vi "HeatingRate.vi"() -> ()   [LabVIEW 2012]
uses:
  <vilib>/Utility/error.llb/DialogType.ctl
  <vilib>/DAQmx/write.llb/DAQmx Write (Digital Wfm 1Chan NSamp).vi
  <vilib>/DAQmx/read.llb/DAQmx Read (Counter 1D U32 1Chan NSamp).vi
  <vilib>/DAQmx/create/channels.llb/DAQmx Create Channel (CI-Count Edges).vi
  <vilib>/DAQmx/create/channels.llb/DAQmx Create Channel (DO-Digital Output).vi
  <vilib>/DAQmx/create/channels.llb/DAQmx Create Channel (CO-Pulse Generation-Frequency).vi
  <vilib>/DAQmx/configure/timing.llb/DAQmx Timing (Implicit).vi
  <vilib>/Waveform/DWDTOps.llb/Digital Pattern Generator (Single Value).vi
  <vilib>/Waveform/DWDTOps.llb/DWDT Append Digital Samples.vi
  <vilib>/Waveform/DWDTOps.llb/DWDT Append Digital Signals.vi
  <vilib>/Waveform/DWDTOps.llb/DWDT Digital Size.vi
  <vilib>/DAQmx/configure/timing.llb/DAQmx Timing (Sample Clock).vi
  <vilib>/Waveform/DWDTOps.llb/DWDT Invert Digital.vi
  <vilib>/Waveform/DWDTOps.llb/DWDT Uncompress Digital.vi
  <vilib>/DAQmx/miscellaneous.llb/DAQmx Fill In Error Info.vi
  <resource>/objmgr/daqmx.rc
panel:
  in  "Mechanical Shutter":bool
  in  "Threshold":u32
  in  "Recool Time (ms)":u32=1000
  out "Run No":i32=16
  in  "Clock Rate":dbl=10000.0
  in  "Off Time (s)":dbl=0.5
  out "Waveform Graph":u32[](graph)=[0, 0, 0, 0, 0, 0, 0, 0, 0, 0, 0, 0, 0, 0, 0, 0, 0, 0, 0, 0, 0, 0, 0, 0, 0, 0, 0, 0, 0, 0, 0, 0, 0, 0, 0, 0, 0, 0, 0, 0, 0, 0, 0, 0, 0, 0, 0, 0, 0, 0, 0, 0, 0, 0, 0, 0, 0, 0, 0, 0, 0, 0, 0, 0, 0, 0, 0, 0, 0, 0, 0, 0, 0, 0, 0, 0, 0, 0, 0, 0, 0, 0, 0, 0, 0, 0, 0, 0, 0, 0, 0, 0, 0, 0, 0, 0, 0, 0, 0, 0, 0, 0, 0, 0, 0, 0, 0, 0, 0, 0, 0, 0, 0, 0, 0, 0, 0, 0, 0, 0, 0, 0, 0, 0, 0, 0, 0, 0, 0, 0, 0, 0, 0, 0, 0, 0, 0, 0, 0, 0, 0, 0, 0, 0, 0, 0, 0, 0, 0, 0, 0, 0, 0, 0, 0, 0, 0, 0, 0, 0, 0, 0, 0, 0, 0, 0, 0, 0, 0, 0, 0, 0, 0, 0, 0, 0, 0, 0, 0, 0, 0, 0, 0, 0, 0, 0, 0, 0, 0, 0, 0, 0, 0, 0, 0, 0, 0, 0, 0, 0, 1, 1, 0, 0, 1, 0, 0, 0, 2, 3, 0, 0, 1, 3, 1, 2, 1, 2, 3, 0, 2, 2, 1, 1, 0, 1, 2, 0, 1, 1, 2, 2, 1, 1, 2, 1, 2, 0, 1, 1, 4, 0, 0, 1, 1, 0, 1, 0, 0, 0, 2, 0, 1, 0, 0, 1, 0, 0, 1, 0, 1, 1, 0, 1, 2, 0, 1, 1, 0, 1, 1, 1, 1, 2, 1, 0, 1, 0, 1, 1, 1, 1, 0, 1, 1, 1, 2, 1, 1, 1, 1, 0, 2, 0, 0, 0, 0, 3, 1, 2, 0, 1, 3, 0, 2, 1, 2, 2, 0, 1, 3, 1, 0, 1, 0, 3, 0, 3, 2, 0, 0, 4, 0, 0, 0, 1, 1, 3, 1, 0, 0, 1, 0, 0, 0, 0, 0, 0, 1, 1, 0, 1, 0, 0, 0, 1, 0, 0, 2, 0, 0, 1, 1, 1, 0, 1, 1, 0, 1, 1, 1, 2, 0, 0, 3, 1, 1, 0, 2, 0, 1, 0, 0, 1, 0, 3, 0, 4, 2, 1, 1, 1, 2, 1, 1, 1, 1, 1, 1, 0, 1, 0, 1, 1, 0, 1, 2, 0, 1]
  in  "Runs":i32=100
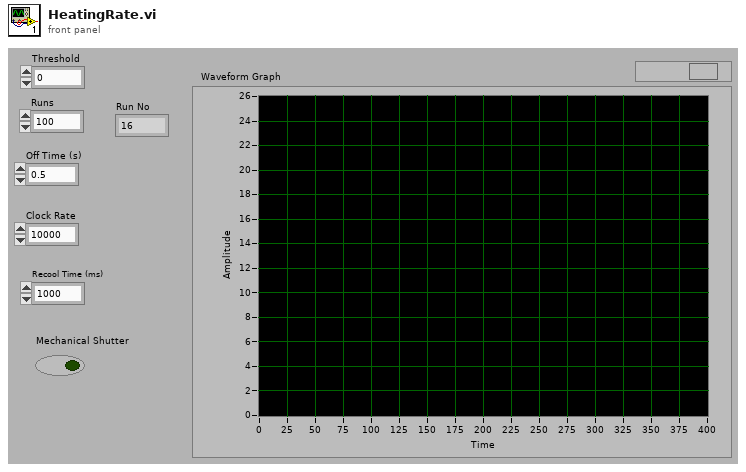
[diagram p1: front panel]
types:
  T1 = enum16{"open", "replace", "create", "open or create", "replace or create", "replace or create with confirmation"}
  T2 = typedef "DialogType.ctl" = u16
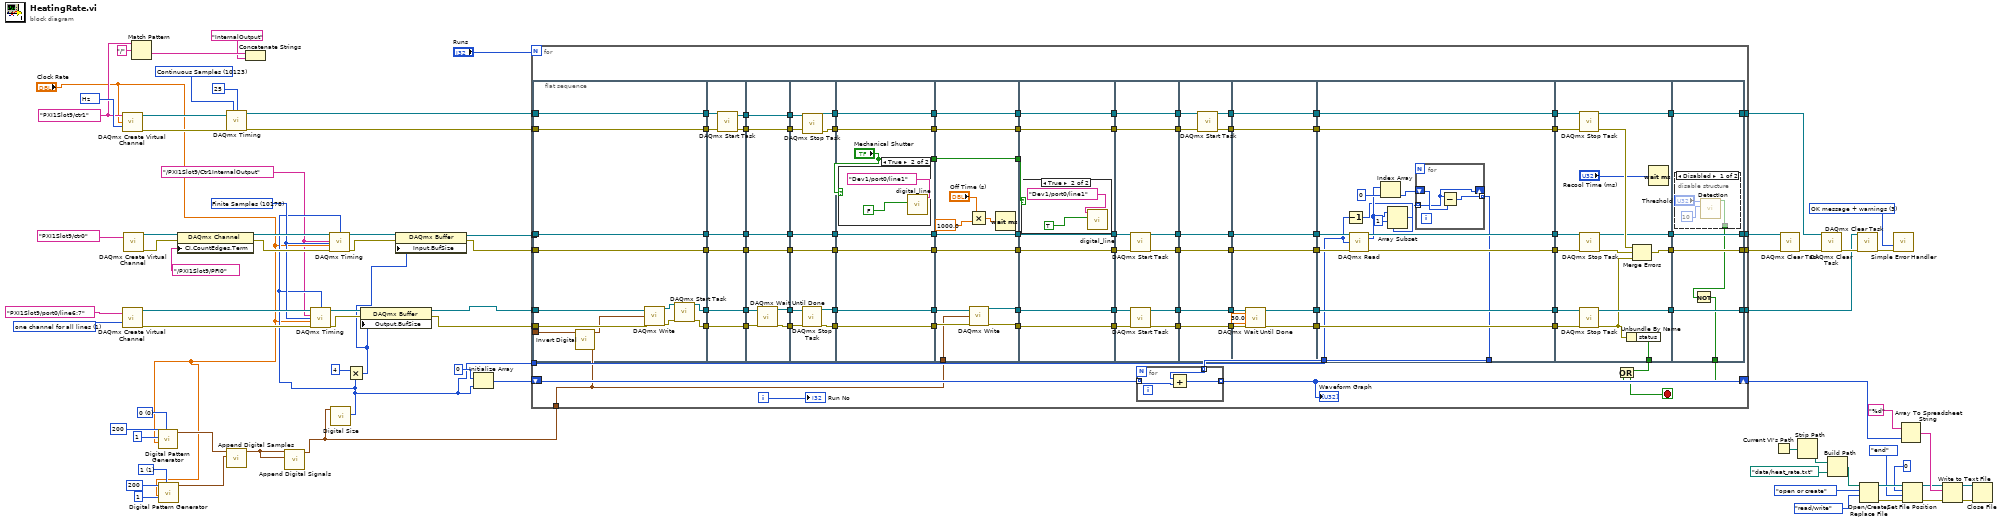
[diagram p0: block diagram]
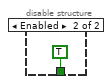
[diagram p4: hidden frame]
diagram:
  w3 = tag "/PXI1Slot9/Ctr1InternalOutput" ("source")
  w16 = u8 1 items=["0", "1", "Z", "L", "H", "X", "T", "V"] ("value")
  w17 = u8 0 items=["0", "1", "Z", "L", "H", "X", "T", "V"] ("value")
  w39 = 10178 items=["Finite Samples"=10178, "Continuous Samples"=10123, "Hardware Timed Single Point"=12522] ("sample mode")
  w52 = T2 3 items=["no dialog", "OK message", "continue or stop message", "OK message + warnings", "continue/stop + warnings"] ("type of dialog (OK msg:1)")
  w58 = 1 items=["one channel for each line", "one channel for all lines"] ("line grouping")
  w61 = tag "PXI1Slot9/ctr1" ("counter")
  w62 = 10373 items=["Hz"=10373] ("units")
  w56 = 10123 items=["Finite Samples"=10178, "Continuous Samples"=10123] ("sample mode")
  n1 = call-poly <vilib>:"DAQmx Create Virtual Channel.vi"("frequency"="Clock Rate", "counter"=w61, "units"=w62) -> ("task out"=w67:refnum<k21>, "error out"=w66:errorcluster)  [unwired: 11 in]
  n2 = call-poly <vilib>:"DAQmx Create Virtual Channel.vi"("lines"=tag "PXI1Slot9/port0/line6:7", "line grouping"=w58) -> ("task out"=w60:refnum<k21>, "error out"=w59:errorcluster)  [unwired: 12 in]
  n3 = call-poly <vilib>:"DAQmx Create Virtual Channel.vi"("counter"=tag "PXI1Slot9/ctr0") -> ("task out"=w70:refnum<k21>, "error out"=w69:errorcluster)  [unwired: 13 in]
  n4 = Match Pattern(string=w61, regular expression="/") -> (after substring=w64:string)  [unwired: 1 in, 3 out]
  n5 = call-poly <vilib>:"Digital Pattern Generator.vi"("value"=w17, "sample rate"="Clock Rate", "number of signals"=u32 1, "number of samples"=u32 200) -> ("digital waveform"=w12:digitalwaveform)  [unwired: 6 in, 1 out]
  n6 = call-poly <vilib>:"Digital Pattern Generator.vi"("value"=w16, "sample rate"="Clock Rate", "number of signals"=u32 1, "number of samples"=u32 200) -> ("digital waveform"=w11:digitalwaveform)  [unwired: 6 in, 1 out]
  n7 = property class="DAQmx Channel"(reference=w70, error in=w69, "CI.CountEdges.Term"=tag "/PXI1Slot9/PFI0") -> (reference out=w72:refnum<k21>, error out=w71:errorcluster)
  n8 = call-poly <vilib>:"DAQmx Timing.vi"("task/channels in"=w67, "sample mode"=w56, "samples per channel"=25, "error in"=w66) -> ("task out"=w2:refnum<k21>, "error out"=w1:errorcluster)  [unwired: 10 in]
  n9 = call-poly <vilib>:"Append Digital Samples.vi"("digital waveform B"=w11, "digital waveform A"=w12) -> ("digital waveform out"=w5:digitalwaveform)  [unwired: 8 in, 1 out]
  n10 = Concatenate Strings(w64, "InternalOutput" ("Local Terminal Name")) -> ()  [unwired: 1 out]
  n11 = call-poly <vilib>:"Append Digital Signals.vi"("digital waveform (low bits)"=w5, "digital waveform (high bits)"=w5) -> ("digital waveform out"=w4:digitalwaveform)  [unwired: 8 in, 1 out]
  n12 = call-poly <vilib>:"Digital Size.vi"("digital waveform in"=w4) -> ("number of samples"=w10:i32)  [unwired: 7 in, 3 out]
  n13 = call-poly <vilib>:"DAQmx Timing.vi"("task/channels in"=w60, "sample mode"=w39, "samples per channel"=w10, "rate"="Clock Rate", "source"=w3, "error in"=w59) -> ("task out"=w47:refnum<k21>, "error out"=w46:errorcluster)  [unwired: 8 in]
  n14 = call-poly <vilib>:"DAQmx Timing.vi"("task/channels in"=w72, "sample mode"=w39, "samples per channel"=w10, "rate"="Clock Rate", "source"=w3, "error in"=w71) -> ("task out"=w44:refnum<k21>, "error out"=w43:errorcluster)  [unwired: 8 in]
  n15 = Multiply(x=4, y=w10) -> (x*y=w18:i32)
  n16 = property class="DAQmx Buffer"(reference=w47, error in=w46, "Output.BufSize"=w18) -> (reference out=w8:refnum<k21>, error out=w7:errorcluster)
  n17 = property class="DAQmx Buffer"(reference=w44, error in=w43, "Input.BufSize"=w18) -> (reference out=w42:refnum<k21>, error out=w41:errorcluster)
  n18 = Initialize Array(0, w10) -> (w38:i32[])
  n19 = for {
    N: "Runs" -> [_]
    tunnel: w8 -> [w140]
    tunnel: w7 -> [w139]
    tunnel: w2 -> [w138]
    tunnel: w1 -> [w137]
    tunnel: [w136] -> w51
    tunnel: [w135] -> w50
    tunnel: [w134] -> w49
    tunnel: [w133] -> w48
    tunnel: w42 -> [w132]
    tunnel: w41 -> [w131]
    shift-right: [w128] -> w33
    shift-left: w38 -> [w130]
    tunnel: w10 -> [w127]
    tunnel: w4 -> [w107]
    i -> [w126]
    stop <- w76 stop-if-true
    n20 = flat-sequence {
      tunnel: w137 -> [w176]
      tunnel: w138 -> [w177]
      tunnel: w139 -> [w174]
      tunnel: w140 -> [w175]
      tunnel: w131 -> [w178]
      tunnel: w132 -> [w179]
      tunnel: [w179] -> w125
      tunnel: [w178] -> w124
      tunnel: [w170] -> w123
      tunnel: [w171] -> w122
      tunnel: [w177] -> w121
      tunnel: [w176] -> w120
      tunnel: w107 -> [w169]
      tunnel: w125 -> [w187]
      tunnel: [w187] -> w119
      tunnel: w124 -> [w186]
      tunnel: [w186] -> w117
      tunnel: w123 -> [w185]
      tunnel: [w185] -> w115
      tunnel: w122 -> [w184]
      tunnel: [w184] -> w113
      tunnel: w121 -> [w183]
      tunnel: w120 -> [w182]
      tunnel: [w181] -> w111
      tunnel: [w180] -> w110
      tunnel: w119 -> [w195]
      tunnel: [w195] -> w118
      tunnel: w117 -> [w194]
      tunnel: [w194] -> w116
      tunnel: w115 -> [w191]
      tunnel: [w190] -> w114
      tunnel: w113 -> [w188]
      tunnel: [w193] -> w112
      tunnel: w111 -> [w193]
      tunnel: w110 -> [w192]
      tunnel: [w192] -> w109
      tunnel: [w189] -> w108
      tunnel: w118 -> [w205]
      tunnel: [w205] -> w106
      tunnel: w116 -> [w204]
      tunnel: [w204] -> w104
      tunnel: w114 -> [w199]
      tunnel: [w196] -> w102
      tunnel: w112 -> [w203]
      tunnel: w109 -> [w202]
      tunnel: w108 -> [w198]
      tunnel: [w201] -> w100
      tunnel: [w200] -> w98
      tunnel: [w197] -> w96
      tunnel: w106 -> [w212]
      tunnel: [w212] -> w105
      tunnel: w104 -> [w211]
      tunnel: [w211] -> w103
      tunnel: w102 -> [w210]
      tunnel: [w210] -> w101
      tunnel: w100 -> [w209]
      tunnel: [w209] -> w99
      tunnel: w98 -> [w208]
      tunnel: [w208] -> w97
      tunnel: w96 -> [w207]
      tunnel: [w207] -> w95
      tunnel: ["Mechanical Shutter"] -> w74
      tunnel: [w227] -> w94
      tunnel: [w226] -> w92
      tunnel: [w217] -> w90
      tunnel: [w218] -> w88
      tunnel: [w225] -> w86
      tunnel: [w224] -> w84
      tunnel: w105 -> [w227]
      tunnel: w103 -> [w226]
      tunnel: w101 -> [w220]
      tunnel: w107 -> [w216]
      tunnel: w99 -> [w225]
      tunnel: w97 -> [w224]
      tunnel: w95 -> [w219]
      tunnel: [w215] -> w75
      tunnel: w74 -> [w215]
      tunnel: w94 -> [w234]
      tunnel: [w234] -> w93
      tunnel: w92 -> [w233]
      tunnel: [w233] -> w91
      tunnel: w90 -> [w232]
      tunnel: [w232] -> w89
      tunnel: w88 -> [w231]
      tunnel: [w231] -> w87
      tunnel: w86 -> [w230]
      tunnel: [w230] -> w85
      tunnel: w84 -> [w229]
      tunnel: [w229] -> w83
      tunnel: w75 -> [w228]
      tunnel: [w242] -> w164
      tunnel: [w241] -> w163
      tunnel: [w240] -> w162
      tunnel: [w239] -> w161
      tunnel: [w238] -> w160
      tunnel: [w237] -> w159
      tunnel: w93 -> [w246]
      tunnel: w91 -> [w245]
      tunnel: w89 -> [w244]
      tunnel: w87 -> [w243]
      tunnel: w85 -> [w242]
      tunnel: w83 -> [w241]
      tunnel: w164 -> [w254]
      tunnel: w163 -> [w253]
      tunnel: [w252] -> w158
      tunnel: w162 -> [w252]
      tunnel: [w251] -> w157
      tunnel: w161 -> [w251]
      tunnel: [w250] -> w156
      tunnel: w160 -> [w250]
      tunnel: [w249] -> w155
      tunnel: w159 -> [w249]
      tunnel: [w248] -> w154
      tunnel: [w247] -> w153
      tunnel: [w263] -> w152
      tunnel: w158 -> [w263]
      tunnel: [w262] -> w151
      tunnel: w157 -> [w262]
      tunnel: w156 -> [w261]
      tunnel: w155 -> [w260]
      tunnel: [w259] -> w150
      tunnel: [w258] -> w149
      tunnel: [w257] -> w148
      tunnel: w154 -> [w257]
      tunnel: [w256] -> w147
      tunnel: w153 -> [w256]
      tunnel: w152 -> [w279]
      tunnel: w151 -> [w278]
      tunnel: [w277] -> w146
      tunnel: [w276] -> w145
      tunnel: [w275] -> w144
      tunnel: w150 -> [w275]
      tunnel: [w274] -> w143
      tunnel: w149 -> [w274]
      tunnel: [w273] -> w142
      tunnel: w148 -> [w273]
      tunnel: [w272] -> w141
      tunnel: w147 -> [w272]
      tunnel: [w265] -> w129
      tunnel: w127 -> [w264]
      tunnel: w146 -> [w297]
      tunnel: w145 -> [w296]
      tunnel: w144 -> [w295]
      tunnel: w143 -> [w294]
      tunnel: w142 -> [w293]
      tunnel: w141 -> [w292]
      tunnel: [w284] -> w78
      tunnel: [w289] -> w82
      tunnel: [w288] -> w81
      tunnel: [w287] -> w80
      tunnel: [w286] -> w79
      tunnel: [w300] -> w133
      tunnel: [w301] -> w134
      tunnel: [w302] -> w135
      tunnel: [w303] -> w136
      tunnel: w82 -> [w303]
      tunnel: w81 -> [w302]
      tunnel: w80 -> [w301]
      tunnel: w79 -> [w300]
      tunnel: [w298] -> w77
      frame #0 {
        n21 = call-poly <vilib>:"Invert Digital.vi"("digital waveform"=w169) -> ("inverted waveform"=w168:digitalwaveform)  [unwired: 9 in, 1 out]
        n22 = call-poly <vilib>:"DAQmx Write.vi"("task/channels in"=w175, "data"=w168, "error in"=w174) -> ("task out"=w173:refnum<k21>, "error out"=w172:errorcluster)  [unwired: 10 in, 1 out]
        n23 = call <vilib>:"DAQmx Start Task.vi"("task/channels in"=w173, "error in"=w172) -> ("task out"=w170:refnum<k21>, "error out"=w171:errorcluster)  [unwired: 12 in]
      }
      frame #1 {
        n24 = call <vilib>:"DAQmx Start Task.vi"("task/channels in"=w183, "error in"=w182) -> ("task out"=w180:refnum<k21>, "error out"=w181:errorcluster)  [unwired: 12 in]
      }
      frame #2 {
        n25 = call <vilib>:"DAQmx Wait Until Done.vi"("task/channels in"=w191, "error in"=w188) -> ("task out"=w190:refnum<k21>, "error out"=w189:errorcluster)  [unwired: 12 in]
      }
      frame #3 {
        n26 = call <vilib>:"DAQmx Stop Task.vi"("task/channels in"=w199, "error in"=w198) -> ("task out"=w196:refnum<k21>, "error out"=w197:errorcluster)  [unwired: 12 in]
        n27 = call <vilib>:"DAQmx Stop Task.vi"("task/channels in"=w202, "error in"=w203) -> ("task out"=w201:refnum<k21>, "error out"=w200:errorcluster)  [unwired: 12 in]
      }
      frame #4 {
        n28 = case shown="True" "Mechanical Shutter" {
          frame False {
          }
          frame True {
            n29 = call "digital_line.vi"("Boolean"=FALSE ("NewVal"), "lines"=tag "Dev1/port0/line1") -> ()  [unwired: 5 in, 1 out]
          }
        }
      }
      frame #5 {
        n30 = Multiply(x="Off Time (s)", y=1000.0) -> (x*y=w221:dbl)
        n31 = call-poly <vilib>:"DAQmx Write.vi"("task/channels in"=w220, "data"=w216, "error in"=w219) -> ("task out"=w217:refnum<k21>, "error out"=w218:errorcluster)  [unwired: 10 in, 1 out]
        n32 = Wait (ms)(milliseconds to wait=w221) -> ()  [unwired: 1 out]
      }
      frame #6 {
        n33 = case shown="True" w228 {
          frame False {
          }
          frame True {
            n34 = call "digital_line.vi"("Boolean"=TRUE ("NewVal"), "lines"=tag "Dev1/port0/line1") -> ()  [unwired: 5 in, 1 out]
          }
        }
      }
      frame #7 {
        n35 = call <vilib>:"DAQmx Start Task.vi"("task/channels in"=w246, "error in"=w245) -> ("task out"=w240:refnum<k21>, "error out"=w239:errorcluster)  [unwired: 12 in]
        n36 = call <vilib>:"DAQmx Start Task.vi"("task/channels in"=w244, "error in"=w243) -> ("task out"=w238:refnum<k21>, "error out"=w237:errorcluster)  [unwired: 12 in]
      }
      frame #8 {
        n37 = call <vilib>:"DAQmx Start Task.vi"("task/channels in"=w254, "error in"=w253) -> ("task out"=w248:refnum<k21>, "error out"=w247:errorcluster)  [unwired: 12 in]
      }
      frame #9 {
        n38 = call <vilib>:"DAQmx Wait Until Done.vi"("task/channels in"=w261, "timeout (sec)"=30.0, "error in"=w260) -> ("task out"=w258:refnum<k21>, "error out"=w259:errorcluster)  [unwired: 11 in]
      }
      frame #10 {
        n39 = Decrement(x=w264) -> (x-1=w267:i32)
        n40 = call-poly <vilib>:"DAQmx Read.vi"("task/channels in"=w279, "number of samples per channel"=w264, "error in"=w278) -> ("task out"=w276:refnum<k21>, "data"=w269:u32[], "error out"=w277:errorcluster)  [unwired: 10 in]
        n41 = Index Array(array=w269, index=0) -> (element=w270:u32)
        n42 = Array Subset(array=w269, index=1, length=w267) -> (w266:u32[])
        n43 = for {
          tunnel: [w282] -> w265 mode=indexing
          shift-right: [w280] -> _
          shift-left: w270 -> [w281]
          tunnel: w266 -> [w280] mode=indexing
          n44 = Subtract(x=w280, y=w281) -> (x-y=w282:u32)
        }
      }
      frame #11 {
        n45 = call <vilib>:"DAQmx Stop Task.vi"("task/channels in"=w293, "error in"=w292) -> ("task out"=w287:refnum<k21>, "error out"=w291:errorcluster)  [unwired: 12 in]
        n46 = call <vilib>:"DAQmx Stop Task.vi"("task/channels in"=w294, "error in"=w295) -> ("task out"=w286:refnum<k21>, "error out"=w285:errorcluster)  [unwired: 12 in]
        n47 = call <vilib>:"DAQmx Stop Task.vi"("task/channels in"=w296, "error in"=w297) -> ("task out"=w288:refnum<k21>, "error out"=w290:errorcluster)  [unwired: 12 in]
        n48 = Unbundle By Name(w285) -> ("status"=w284:bool)
        n49 = Merge Errors(w291, w290, w285) -> (w289:errorcluster)
        n50 = Wait (ms)(milliseconds to wait="Recool Time (ms)") -> ()  [unwired: 1 out]
      }
      frame #12 {
        n51 = disable-structure shown="Disabled" {
          disable-tunnel: [w304 TRUE ("Ion")] -> w299
          frame Disabled {
            n52 = call "DetectIon.vi"("Samples per averaging\nblock"=10 ("Samples per averaging\nblock"), "Threshold"="Threshold") -> ("Ion"=w304:bool)  [unwired: 9 in]
          }
          frame Enabled {
          }
        }
        n53 = Not(x=w299) -> (.not. x?=w298:bool)
      }
    }
    n54 = for {
      tunnel: w130 -> [w167] mode=indexing
      tunnel: w129 -> [w166] mode=indexing
      tunnel: [w165] -> w128 mode=indexing
      n55 = Add(x=w166, y=w167) -> (x+y=w165:u32)
    }
    "Waveform Graph" <- w128
    n56 = Or(x=w78, y=w77) -> (x .or. y?=w76:bool)
    "Run No" <- w126
  }
  n57 = Current VI's Path() -> (path=w27:path)
  n58 = call <vilib>:"DAQmx Clear Task.vi"("task in"=w50, "error in"=w51) -> ("error out"=w55:errorcluster)  [unwired: 13 in]
  n59 = Strip Path(path=w27) -> (stripped path=w26:path)  [unwired: 1 out]
  n60 = call <vilib>:"DAQmx Clear Task.vi"("task in"=w49, "error in"=w55) -> ("error out"=w54:errorcluster)  [unwired: 13 in]
  n61 = Build Path(base path=w26, name or relative path=path "data/heat_rate.txt" ("file path (use dialog)")) -> (appended path=w28:path)
  n62 = call <vilib>:"DAQmx Clear Task.vi"("task in"=w48, "error in"=w54) -> ("error out"=w53:errorcluster)  [unwired: 13 in]
  n63 = Open/Create/Replace File(file path (use dialog)=w28, operation (0:open)=T1."open or create", access (0:read/write)=enum16{"read/write", "read-only", "write-only"}."read/write") -> (refnum out=w24:refnum<file>, error out=w25:errorcluster)  [unwired: 3 in, 1 out]
  n64 = call <vilib>:"Simple Error Handler.vi"("type of dialog (OK msg:1)"=w52, "error in (no error)"=w53) -> ()  [unwired: 3 in, 5 out]
  n65 = Array To Spreadsheet String(array=w33, 3:"%d" ("format string")) -> (spreadsheet string=w32:string)  [unwired: 1 in]
  n66 = Set File Position(offset (in bytes) (0)=i64 0, refnum=w24, from (0:start)=enum16{"start", "end", "current"}."end", error in=w25) -> (refnum out=w22:refnum<file>, error out=w23:errorcluster)
  n67 = Write to Text File(file (use dialog)=w22, text=w32, error in=w23) -> (refnum out=w31:refnum<file>, error out=w30:errorcluster)  [unwired: 1 in, 1 out]
  n68 = Close File(refnum=w31, error in=w30) -> ()  [unwired: 2 out]
